vi "SentenceFromFile (SubVI).vi"(8 "error in (no error)":errorcluster, 10 "UUT":u8) -> (0 "error out":errorcluster, 2 "Sentence":string)   [LabVIEW 2017]
uses:
  <vilib>/Utility/config.llb/Read Key (String).vi
  <vilib>/Utility/config.llb/NI_LVConfig.lvlib
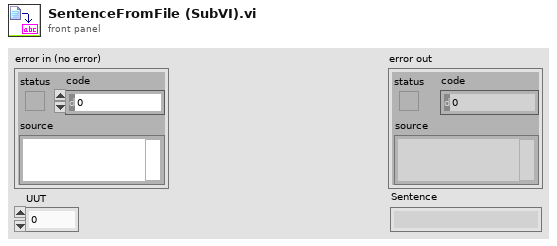
[diagram p1: front panel]
types:
  T1 = typedef "NI_LVConfig.lvlib/Config Data RefNum.ctl" = refnum<k1>
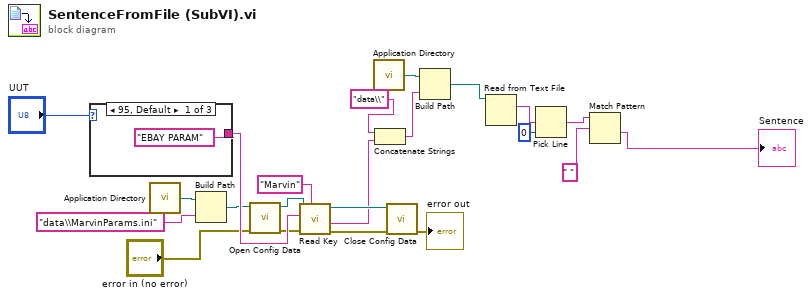
[diagram p0: block diagram]
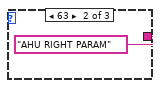
[diagram p2: hidden frame]
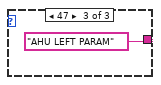
[diagram p3: hidden frame]
diagram:
  n1 = case shown="95, Default" "UUT" {
    tunnel: ["EBAY PARAM" ("section") "AHU RIGHT PARAM" ("section") "AHU LEFT PARAM" ("section")] -> w22
    frame 95, Default {
    }
    frame 63 {
    }
    frame 47 {
    }
  }
  n2 = call <vilib>:"Application Directory.vi"() -> ("Application Directory"=w14:path)
  n3 = Build Path(base path=w14, name or relative path="data\\MarvinParams.ini") -> (appended path=w18:path)
  n4 = call <vilib>:"Open Config Data.vi"("error in (no error)"="error in (no error)", "configuration file path"=w18) -> ("error out"=w19:errorcluster, "refnum"=w16:T1)  [unwired: 1 in, 7 out]
  n5 = call-poly <vilib>:"Read Key.vi"("section"="Marvin", "error in (no error)"=w19, "key"=w22, "refnum"=w16) -> ("error out"=w20:errorcluster, "value"=w7:string, "refnum out"=w21:T1)  [unwired: 2 in, 3 out]
  n6 = call <vilib>:"Application Directory.vi"() -> ("Application Directory"=w10:path)
  n7 = Concatenate Strings("data\\" ("name or relative path"), w7) -> (w8:string)
  n8 = call <vilib>:"Close Config Data.vi"("error in (no error)"=w20, "refnum"=w21) -> ("error out"=→"error out":errorcluster)  [unwired: 8 in, 1 out]
  n9 = Build Path(base path=w10, name or relative path=w8) -> (appended path=w6:path)
  n10 = Read from Text File(file (use dialog)=w6) -> (text=w4:string)  [unwired: 3 in, 3 out]
  n11 = Pick Line(multi-line string=w4, line index=0) -> (output string=w3:string)  [unwired: 1 in]
  n12 = Match Pattern(string=w3, regular expression=" ") -> (after substring=→"Sentence":string)  [unwired: 1 in, 3 out]
